vi "amplitude threshold input (SubVI).vi"(9 "threshold":dbl, 10 "%max amplitude":dbl, 11 "Array":dbl[](array[numeric])) -> (2 "actual ratio (%)":dbl, 3 "Index":i32)   [LabVIEW 2012]
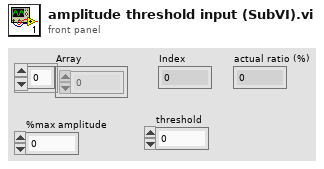
[diagram p1: front panel]
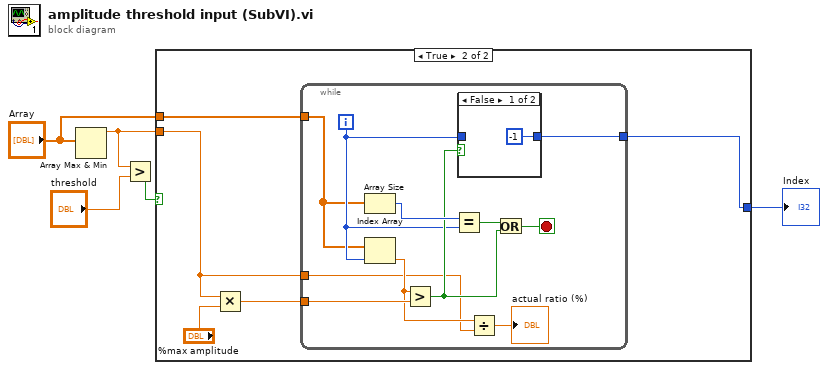
[diagram p0: block diagram]
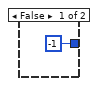
[diagram p2: hidden frame]
diagram:
  n1 = Array Max & Min(array="Array") -> (max value=w2:dbl)  [unwired: 3 out]
  n2 = Greater?(x=w2, y="threshold") -> (0:w3:bool)
  n3 = case shown="True" w3 {
    tunnel: [-1 w11] -> w5
    tunnel: w2 -> [_ w7]
    tunnel: "Array" -> [_ w9]
    frame False {
    }
    frame True {
      n4 = Multiply(x=w7, y="%max amplitude") -> (x*y=w8:dbl)
      n5 = while {
        tunnel: [w17] -> w11
        tunnel: w9 -> [w16]
        tunnel: w8 -> [w15]
        tunnel: w7 -> [w13]
        i -> [w18]
        stop <- w21 stop-if-true
        n6 = Array Size(array=w16) -> (size(s)=w22:i32)
        n7 = Index Array(array=w16, index=w18) -> (element=w14:dbl)
        n8 = Greater?(x=w14, y=w15) -> (0:w19:bool)
        n9 = Equal?(x=w22, y=w18) -> (x = y?=w20:bool)
        n10 = case shown="False" w19 {
          tunnel: w18 -> [_ w24]
          tunnel: [-1 w24] -> w17
          frame False {
          }
          frame True {
          }
        }
        n11 = Divide(x=w14, y=w13) -> (x/y=→"actual ratio (%)":dbl)
        n12 = Or(x=w20, y=w19) -> (x .or. y?=w21:bool)
      }
    }
  }
  "Index" <- w5
